vi "SetGageConfig.vi"(10 "Gage Acqu.":T4, 11 "Handle Cluster":T5) -> ()   [LabVIEW 2013]
uses:
  <vilib>/Utility/error.llb/DialogType.ctl
  GageAcqu.Refs.ctl
panel:
  in  "Trigger":T1={"Slope"=0, "Level"=0, "Source"=0, "External Range"=2000, "External Coupling"=0, "External"=TRUE, "Disable"=FALSE, "External Impedance"=0} {"External Impedance" items=["50 Ohm", "HiZ"]; "External Coupling" items=["DC", "AC"]; "External Range" min=2000 max=10000 step=8000; "Slope" items=["Rising", "Falling"]; "Level" min=-100 max=100; "Source" min=0 max=64 step=1}
  in  "Acquisition":T2={"Sample Rate"=100000000.0, "Mode"=1, "Depth"=8192.0, "Segment Size"=8192.0, "Trigger Timeout"=1000000.0, "Trigger Holdoff"=0.0, "Trigger Delay"=0.0, "Clock mode"=enum."Internal"} {"Segment Size" min=256.0 step=128.0; "Trigger Delay" min=0.0 step=128.0; "Trigger Timeout" format="%.0p"; "Trigger Holdoff" min=0.0 step=128.0; "Depth" min=256.0 step=128.0; "Mode" items=["Single", "Dual", "Quad", "Octal"]; "Sample Rate" format="%.0p"}
  in  "Channels":T3(array[cluster])=[{"Coupling"=0, "Differential Input"=FALSE, "Direct-to-ADC"=FALSE, "Range"=2000, "Impedance"=50, "DC Offset"=0, "Filter"=0}, {"Coupling"=0, "Differential Input"=FALSE, "Direct-to-ADC"=FALSE, "Range"=2000, "Impedance"=50, "DC Offset"=0, "Filter"=0}] {"Impedance" min=50 max=1000000 step=999950; "Coupling" items=["DC", "AC"]}
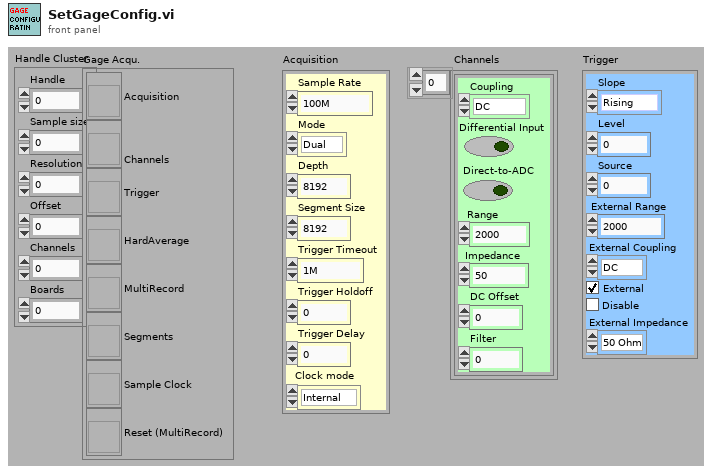
[diagram p1: front panel]
types:
  T1 = cluster{"Slope":u16, "Level":i32, "Source":i32, "External Range":u32, "External Coupling":u16, "External":bool, "Disable":bool, "External Impedance":u16}
  T2 = cluster{"Sample Rate":dbl, "Mode":u16, "Depth":dbl, "Segment Size":dbl, "Trigger Timeout":dbl, "Trigger Holdoff":dbl, "Trigger Delay":dbl, "Clock mode":enum16{"Internal", "External", "Reference"}}
  T3 = cluster{"Coupling":u16, "Differential Input":bool, "Direct-to-ADC":bool, "Range":u32, "Impedance":u32, "DC Offset":i32, "Filter":i32}[]
  T4 = typedef "GageAcqu.Refs.ctl" = cluster{"Acquisition":refnum<vi>, "Channels":refnum<vi>, "Trigger":refnum<vi>, "HardAverage":refnum<vi>, "MultiRecord":refnum<vi>, "Segments":refnum<vi>, "Sample Clock":refnum<vi>, "Reset (MultiRecord)":refnum<vi>}
  T5 = cluster{"Handle":u32, "Sample size":u32, "Resolution":i32, "Offset":i32, "Channels":u32, "Boards":u32}
  T6 = cluster{"Coupling":u16, "Differential Input":bool, "Direct-to-ADC":bool, "Range (mV)":u32, "Impedance":u32, "DC Offset":i32, "Filter":i32}[]
  T7 = cluster{string, "Differential Input":bool, "Direct-to-ADC":bool, "Range (mV)":u32, "Impedance":u32, "DC Offset":i32, "Filter":i32}
  T8 = cluster{"Sample Rate":dbl, "Clock mode":enum16{"Internal", "External", "Reference"}, "RingText.Text":string, "Depth":dbl, "Segment Size":dbl, "Trigger Timeout":dbl, "Trigger Holdoff":dbl, "Trigger Delay":dbl}
  T9 = cluster{void, "Level":i32, "Source":i32, "External Range":u32, void, "External":bool, "Disable":bool, void}
  T10 = cluster{void, "Level":i32, "Source":i32, "External Range":u32, void, "External":bool, "Disable":bool, void}[]
  T11 = typedef "DialogType.ctl" = u16
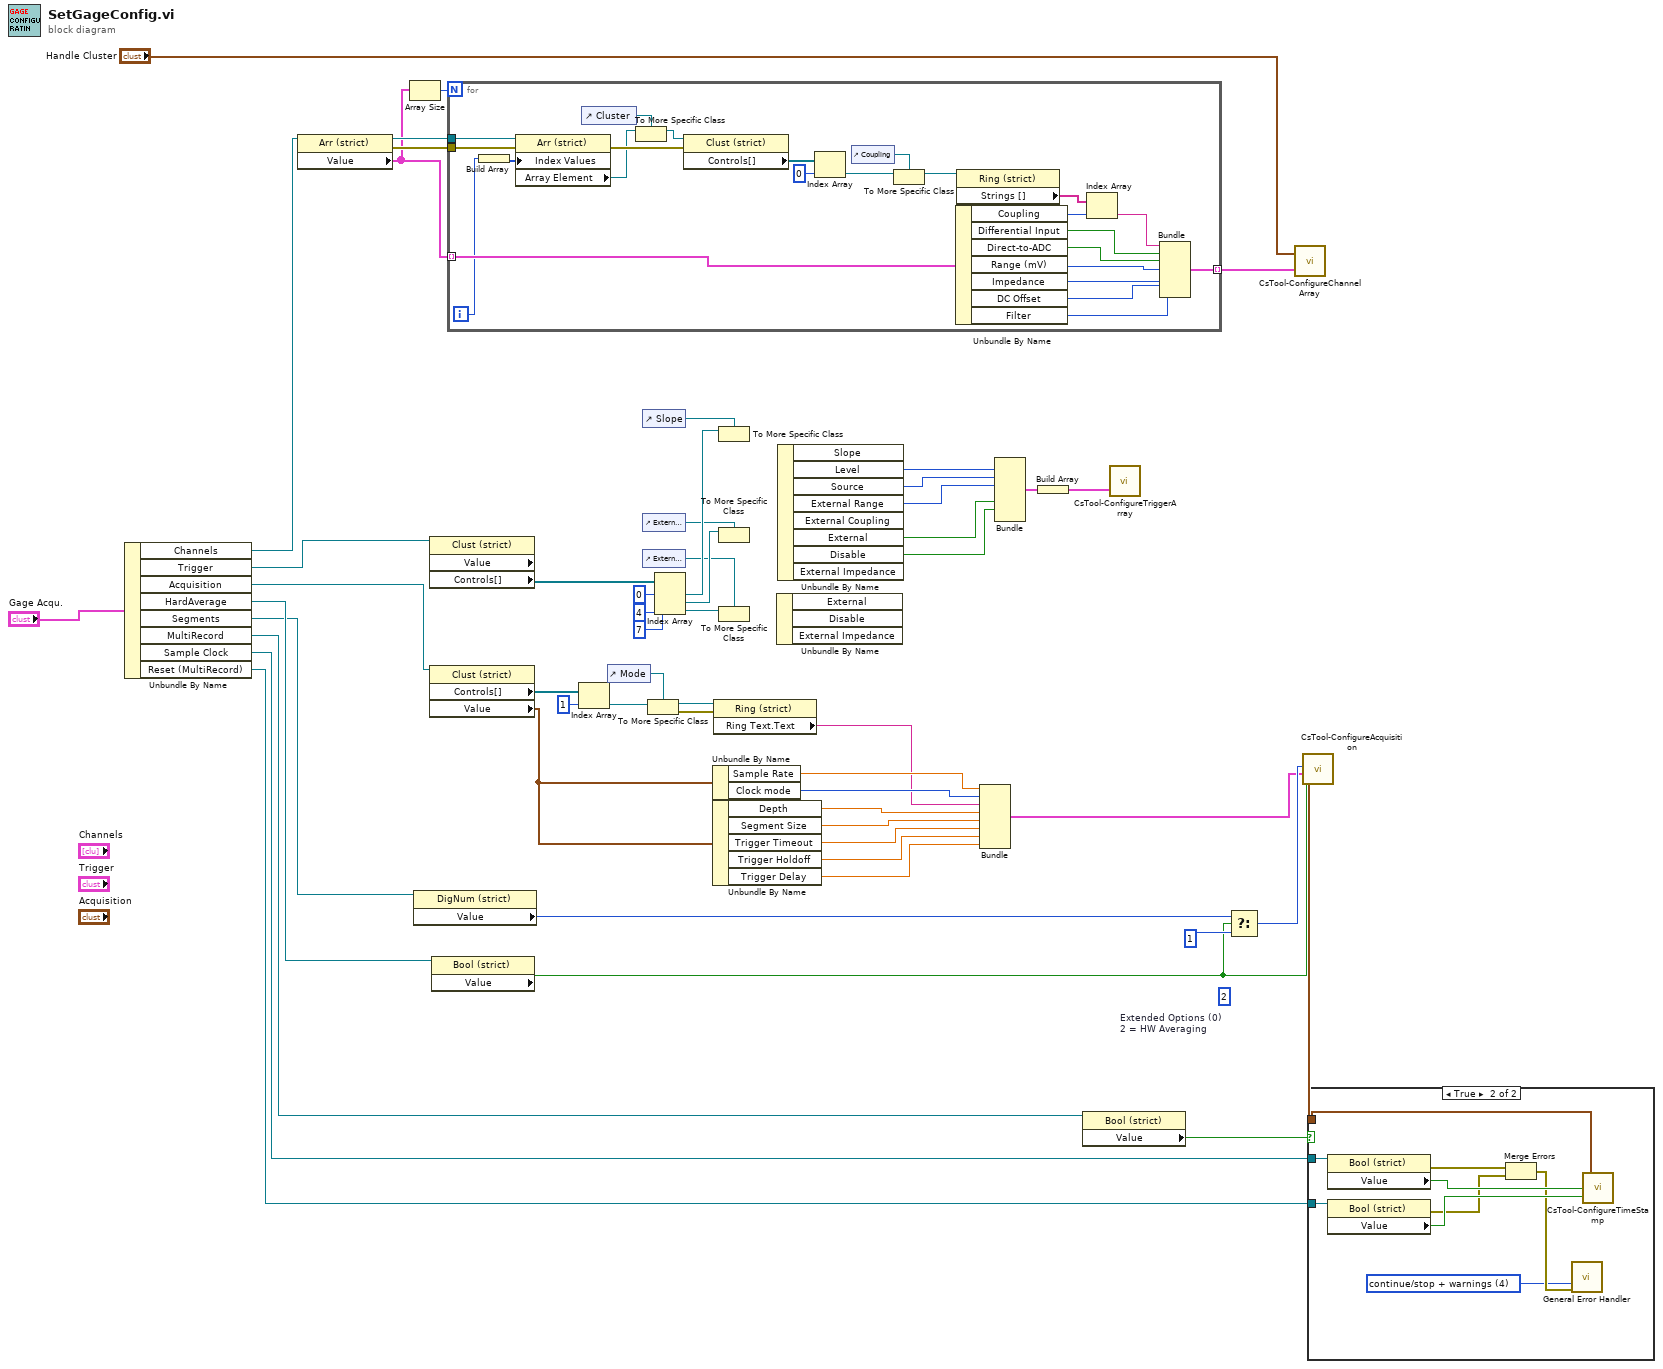
[diagram p0: block diagram]
diagram:
  (unwired) 2  # Extended Options (0) 2 = HW Averaging
  n1 = Unbundle By Name("Gage Acqu.") -> ("Channels"=w54:refnum<vi>, "Trigger"=w53:refnum<vi>, "Acquisition"=w52:refnum<vi>, "HardAverage"=w51:refnum<vi>, "Segments"=w47:refnum<vi>, "MultiRecord"=w6:refnum<vi>, "Sample Clock"=w8:refnum<vi>, "Reset (MultiRecord)"=w7:refnum<vi>)
  n2 = property on="Property Node" class="Arr (strict)"(reference=w54) -> (reference out=w29:refnum<vi>, error out=w28:errorcluster, "Value"=w10:T6)  [unwired: 1 in]
  n3 = Array Size(array=w10) -> (size(s)=w11:i32)
  n4 = property on="Property Node" class="DigNum (strict)"(reference=w47) -> ("Value"=w46:u32)  [unwired: 1 in, 2 out]
  n5 = property on="Property Node" class="Clust (strict)"(reference=w53) -> ("Value"=w41:T1, "Controls[]"=w40:refnum<vi>[])  [unwired: 1 in, 2 out]
  n6 = property on="Property Node" class="Clust (strict)"(reference=w52) -> ("Controls[]"=w17:refnum<vi>[], "Value"=w12:T2)  [unwired: 1 in, 2 out]
  n7 = property on="Property Node" class="Bool (strict)"(reference=w51) -> ("Value"=w48:bool)  [unwired: 1 in, 2 out]
  n8 = for {
    N: w11 -> [_]
    tunnel: w10 -> [w77] mode=indexing
    tunnel: [w78] -> w27 mode=indexing
    tunnel: w29 -> [w69]
    tunnel: w28 -> [w67]
    i -> [w59]
    n9 = Build Array(w59) -> (w58:i32[])
    n10 = property on="Property Node" class="Arr (strict)"(reference=w69, error in=w67, "Index Values"=w58) -> (error out=w68:errorcluster, "Array Element"=w57:refnum<vi>)  [unwired: 1 out]
    n11 = control-ref of="Cluster"() -> (w65:refnum<vi>)
    n12 = To More Specific Class(target class=w65, reference=w57) -> (specific class reference=w66:refnum<vi>)  [unwired: 1 in, 1 out]
    n13 = property on="Property Node" class="Clust (strict)"(reference=w66, error in=w68) -> ("Controls[]"=w64:refnum<vi>[])  [unwired: 2 out]
    n14 = Index Array(array=w64, index=0) -> (element=w62:refnum<vi>)
    n15 = control-ref of="Coupling"() -> (w60:refnum<vi>)
    n16 = To More Specific Class(target class=w60, reference=w62) -> (specific class reference=w61:refnum<vi>)  [unwired: 1 in, 1 out]
    n17 = Unbundle By Name(w77) -> ("Coupling"=w74:u16, "Differential Input"=w79:bool, "Direct-to-ADC"=w73:bool, "Range (mV)"=w72:u32, "Impedance"=w71:u32, "DC Offset"=w70:i32, "Filter"=w56:i32)
    n18 = property on="Property Node" class="Ring (strict)"(reference=w61) -> ("Strings []"=w76:string[])  [unwired: 1 in, 2 out]
    n19 = Index Array(array=w76, index=w74) -> (element=w75:string)
    n20 = Bundle(w75, "Differential Input"=w79, "Direct-to-ADC"=w73, "Range (mV)"=w72, "Impedance"=w71, "DC Offset"=w70, "Filter"=w56) -> (w78:T7)  [unwired: 1 in]
  }
  n21 = Index Array(array=w17, index=1) -> (element=w15:refnum<vi>)
  n22 = control-ref of="Mode"() -> (w14:refnum<vi>)
  n23 = control-ref of="Slope"() -> (w36:refnum<vi>)
  n24 = control-ref of="External Coupling"() -> (w33:refnum<vi>)
  n25 = control-ref of="External Impedance"() -> (w32:refnum<vi>)
  n26 = To More Specific Class(target class=w14, reference=w15) -> (specific class reference=w13:refnum<vi>, error out=w9:errorcluster)  [unwired: 1 in]
  n27 = Index Array(array=w40, index #1=0 ("index"), index #2=4 ("index"), index #3=7 ("index")) -> (element #1=w35:refnum<vi>, element #2=w34:refnum<vi>, element #3=w31:refnum<vi>)
  n28 = Unbundle By Name(w12) -> ("Sample Rate"=w20:dbl, "Clock mode"=w22:enum16{"Internal", "External", "Reference"})
  n29 = Unbundle By Name(w12) -> ("Depth"=w21:dbl, "Segment Size"=w23:dbl, "Trigger Timeout"=w24:dbl, "Trigger Holdoff"=w25:dbl, "Trigger Delay"=w26:dbl)
  n30 = property on="Property Node" class="Ring (strict)"(reference=w13, error in=w9) -> ("Ring Text.Text"=w19:string)  [unwired: 2 out]
  n31 = To More Specific Class(target class=w36, reference=w35) -> ()  [unwired: 1 in, 2 out]
  n32 = To More Specific Class(target class=w33, reference=w34) -> ()  [unwired: 1 in, 2 out]
  n33 = To More Specific Class(target class=w32, reference=w31) -> ()  [unwired: 1 in, 2 out]
  n34 = Unbundle By Name() -> ()  [unwired: 1 in, 3 out]
  n35 = Unbundle By Name() -> ("Level"=w42:i32, "Source"=w43:i32, "External Range"=w44:u32, "External"=w1:bool, "Disable"=w2:bool)  [unwired: 1 in, 3 out]
  n36 = Bundle("Sample Rate"=w20, "Clock mode"=w22, "RingText.Text"=w19, "Depth"=w21, "Segment Size"=w23, "Trigger Timeout"=w24, "Trigger Holdoff"=w25, "Trigger Delay"=w26) -> (w18:T8)  [unwired: 1 in]
  n37 = Bundle("Level"=w42, "Source"=w43, "External Range"=w44, "External"=w1, "Disable"=w2) -> (w30:T9)  [unwired: 4 in]
  n38 = Build Array(w30) -> (w50:T10)
  n39 = property on="Property Node" class="Bool (strict)"(reference=w6) -> ("Value"=w5:bool)  [unwired: 1 in, 2 out]
  n40 = call <instrlib>:"CsTool-ConfigureTriggerArray.vi"("Triggers"=w50) -> ()  [unwired: 1 in, 1 out]
  n41 = Select(t=w46, s=w48, f=u32 1 ("HW Average")) -> (s? t:f=w45:u32)
  n42 = call <instrlib>:"CsTool-ConfigureChannelArray.vi"("Channels"=w27, "Handle Cluster"="Handle Cluster") -> ()  [unwired: 1 out]
  n43 = call <instrlib>:"CsTool-ConfigureAcquisition.vi"("Segment Count (1)"=w45, "Acquisition"=w18, "Invert Clock (f)"=w48) -> ("Handle Cluster"=w3:T5)  [unwired: 1 in, 1 out]
  n44 = case shown="True" w5 {
    tunnel: w8 -> [_ w88]
    tunnel: w7 -> [_ w87]
    tunnel: w3 -> [_ w84]
    frame False {
    }
    frame True {
      w80 = T11 4 items=["no dialog", "OK message", "continue or stop message", "OK message + warnings", "continue/stop + warnings"] ("type of dialog (OK msg:1)")
      n45 = property on="Property Node" class="Bool (strict)"(reference=w88) -> (error out=w83:errorcluster, "Value"=w86:bool)  [unwired: 1 in, 1 out]
      n46 = property on="Property Node" class="Bool (strict)"(reference=w87) -> (error out=w82:errorcluster, "Value"=w85:bool)  [unwired: 1 in, 1 out]
      n47 = Merge Errors(w83, w82) -> (w81:errorcluster)
      n48 = call <vilib>:"General Error Handler.vi"("type of dialog (OK msg:1)"=w80, "error in (no error)"=w81) -> ()  [unwired: 9 in, 5 out]
      n49 = call <instrlib>:"CsTool-ConfigureTimeStamp.vi"("Reset"=w85, "Sample Clock"=w86, "Handle Cluster"=w84) -> ()  [unwired: 1 out]
    }
  }
